vi "Send Email using SMTP Client.vi"(7 "map?":bool, 8 "error in (no error)":errorcluster, 9 "Message":string, 10 "subject":string="\"Hello\" ") -> (0 "error out":errorcluster)   [LabVIEW 2019]
panel:
  out "standard error":string
  out "standard output":string
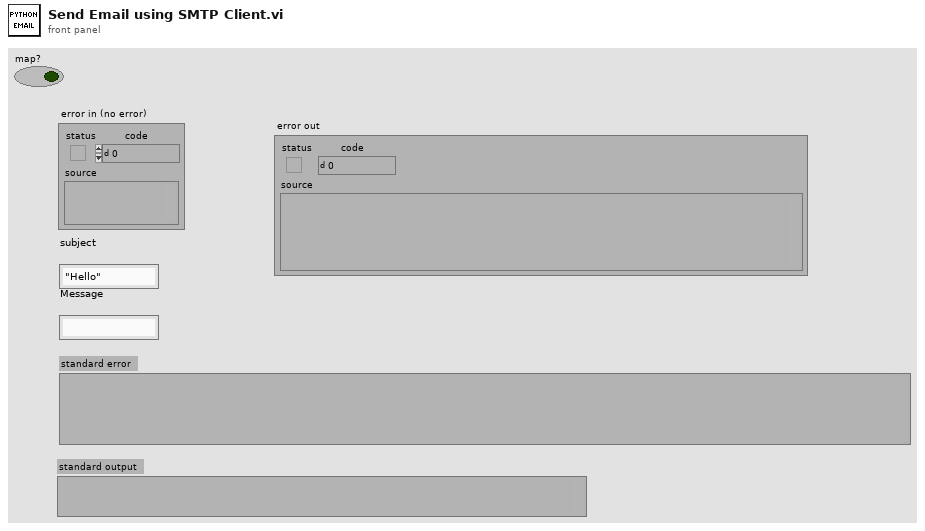
[diagram p1: front panel]
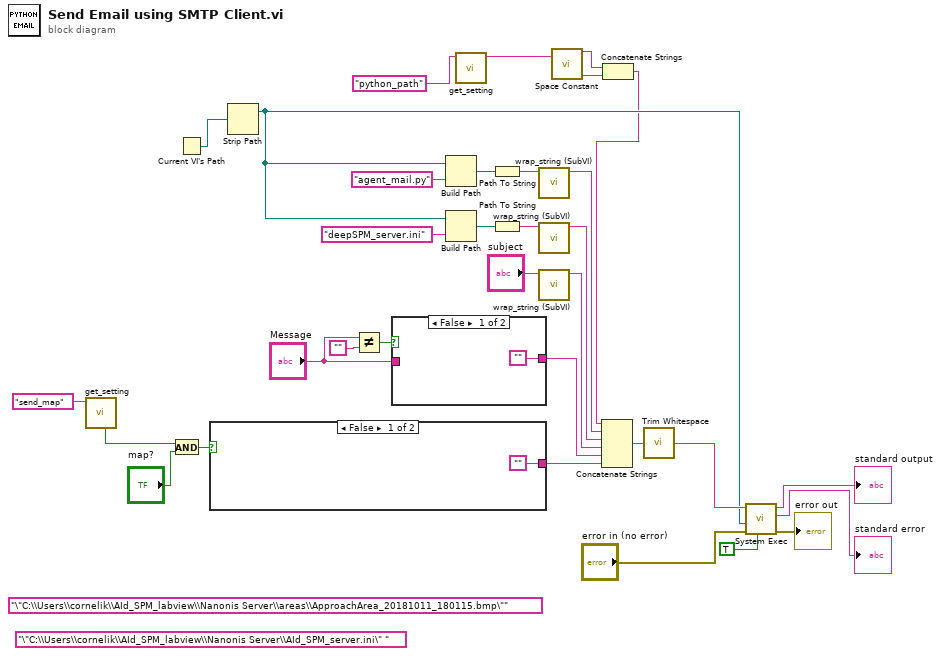
[diagram p0: block diagram]
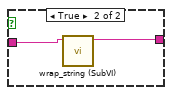
[diagram p2: hidden frame]
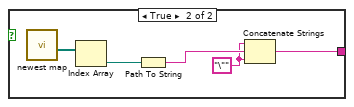
[diagram p3: hidden frame]
diagram:
  (unwired) "\"C:\\Users\\cornelik\\AId_SPM_labview\\Nanonis Server\\areas\\ApproachArea_20181011_180115.bmp\"" ("string")
  (unwired) "\"C:\\Users\\cornelik\\AId_SPM_labview\\Nanonis Server\\AId_SPM_server.ini\" " ("string")
  n1 = call "get_setting.vi"("key"="send_map") -> ("Boolean"=w25:bool)  [unwired: 6 in, 4 out]
  n2 = And(x=w25, y="map?") -> (x .and. y?=w13:bool)
  n3 = Current VI's Path() -> (path=w6:path)
  n4 = case shown="False" w13 {
    tunnel: ["" w34] -> w21
    frame False {
    }
    frame True {
      w37 = "\"" ("string")
      n5 = call "newest map.vi"() -> ("newest map"=w35:path[])  [unwired: 11 in]
      n6 = Index Array(array=w35) -> (element=w36:path)  [unwired: 1 in]
      n7 = Path To String(path=w36) -> (string=w38:string)
      n8 = Concatenate Strings(w37, w38, w37) -> (w34:string)
    }
  }
  n9 = Strip Path(path=w6) -> (stripped path=w5:path)  [unwired: 1 out]
  n10 = Not Equal?(x="Message", y="") -> (x != y?=w9:bool)
  n11 = case shown="False" w9 {
    tunnel: "Message" -> [_ w41]
    tunnel: ["" w40] -> w16
    frame False {
    }
    frame True {
      n12 = call "wrap_string (SubVI).vi"("in"=w41) -> ("String"=w40:string)  [unwired: 10 in]
    }
  }
  n13 = Build Path(base path=w5, name or relative path="agent_mail.py" ("command line")) -> (appended path=w17:path)
  n14 = Build Path(base path=w5, name or relative path="deepSPM_server.ini") -> (appended path=w18:path)
  n15 = call "get_setting.vi"("key"="python_path") -> ("value"=w3:string)  [unwired: 6 in, 4 out]
  n16 = Path To String(path=w17) -> (string=w20:string)
  n17 = Path To String(path=w18) -> (string=w19:string)
  n18 = call "wrap_string (SubVI).vi"("in"=w20) -> ("String"=w22:string)  [unwired: 10 in]
  n19 = call "wrap_string (SubVI).vi"("in"=w19) -> ("String"=w28:string)  [unwired: 10 in]
  n20 = call "wrap_string (SubVI).vi"("in"="subject") -> ("String"=w14:string)  [unwired: 10 in]
  n21 = call <vilib>:"Space Constant.vi"() -> ("String"=w2:string)
  n22 = Concatenate Strings(w3, w2) -> (w1:string)
  n23 = Concatenate Strings(w1, w22, w28, w14, w16, w21) -> (w8:string)
  n24 = call <vilib>:"Trim Whitespace.vi"("string"=w8) -> ("trimmed string"=w7:string)  [unwired: 1 in]
  n25 = call <vilib>:"System Exec.vi"("run minimized? (F)"=TRUE, "error in (no error)"="error in (no error)", "working directory"=w5, "command line"=w7) -> ("error out"=→"error out":errorcluster, "standard error"=→"standard error":string, "standard output"=→"standard output":string)  [unwired: 4 in, 1 out]
